vi "Value Optimize.vi"(8 "error in (no error)":errorcluster caption="错误输入（无错误）", 9 "value":dbl, 10 "optimize":i32, 11 "asicHandle":i32) -> (0 "error out":errorcluster caption="错误输出", 3 "function return":i32)   [LabVIEW 2018]
doc: "extern int __stdcall APSxValueOptimize (int asicHandle, IN int optimize, IN double value);"
uses:
  APSx.dll/APSx.dll
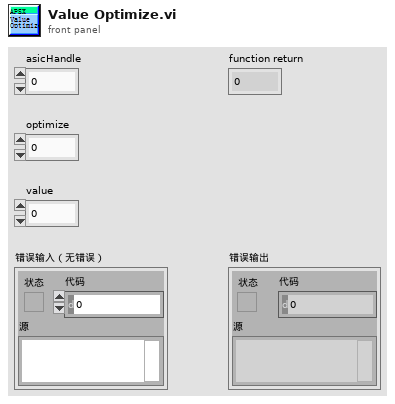
[diagram p1: front panel]
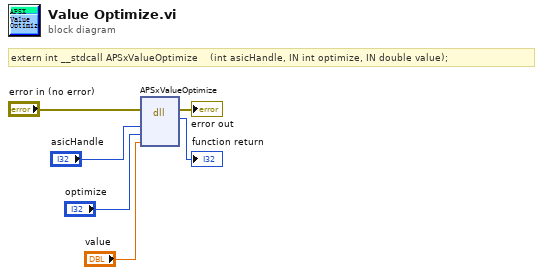
[diagram p0: block diagram]
diagram:
  # "extern int __stdcall APSxValueOptimize    (int asicHandle, IN int optimize, IN double value);"
  n1 = dll-call lib="PTH2[abs D项目Feng恒隆项目Labview传感器对中台SourcesAPSx.dllAPSx.*" fn="APSxValueOptimize"(error in="error in (no error)", "asicHandle"="asicHandle", "optimize"="optimize", "value"="value") -> (error out=→"error out":errorcluster, →"function return":i32)  [unwired: 5 in, 1 out]
